vi "MegaAnalysis5.vi"() -> ()   [LabVIEW 2016]
uses:
  <vilib>/Analysis/4window.llb/windowTd.ctl
  <vilib>/Analysis/Matrix/Datatypes/RealMatrix.ctl
  <vilib>/Analysis/baseanly.llb/Mean (DBL).vi
  <vilib>/Analysis/4window.llb/Hanning Window (DBL).vi
  <vilib>/Analysis/2dsp.llb/Real FFT.vi
  <vilib>/Analysis/2dsp.llb/Inverse Real FFT.vi
  <vilib>/Analysis/4window.llb/AllCosWindow (DBL).vi
  subs/status.vi
  <vilib>/Utility/file.llb/Write To Spreadsheet File (I64).vi
  <vilib>/Utility/file.llb/Write To Spreadsheet File (string).vi
  <vilib>/Utility/file.llb/Read From Spreadsheet File (string).vi
  <vilib>/Utility/file.llb/Read From Spreadsheet File (DBL).vi
  <vilib>/Analysis/3filter.llb/Butterworth Filter (DBL).vi
  <vilib>/Analysis/3filter.llb/Chebyshev Filter (DBL).vi
  <vilib>/Analysis/3filter.llb/Inverse Chebyshev Filter (DBL).vi
  <vilib>/Analysis/3filter.llb/Elliptic Filter (DBL).vi
  <vilib>/Analysis/3filter.llb/Bessel Filter (DBL).vi
  <vilib>/measure/mamon.llb/Waveform Peak Detection for 1 Chan.vi
  <vilib>/Analysis/0measdsp.llb/Scaled Time Domain Window (DBL).vi
  <vilib>/Utility/file.llb/Write To Spreadsheet File (DBL).vi
  <vilib>/Analysis/NI_AALBase.lvlib
  <vilib>/measure/NI_MAPro.lvlib
  <vilib>/gmath/NI_Gmath.lvlib
  <vilib>/Analysis/NI_AALPro.lvlib
  <vilib>/Analysis/Matrix/NI_Matrix.lvlib
panel:
  in  "?":bool
  out "activity":string
  in  "?":bool
  in  "transform:":u16(ring)=3 items=["time", "B", "1/B", "data"]
  in  "?":T1(tab)=enum."data select"
  in  "Notes (saved along with settings)":string
  in  "?":bool
  in  "?":bool
  in  "Base path for data storage":path
  in  "?":bool
  in  "?":bool=TRUE
  in  "?":bool=TRUE
  in  "?":bool
  in  "?":bool=TRUE
  in  "?":bool=TRUE
  in  "?":bool
  in  "skip":u16=1
  in  "?":T2(tab)=enum."assign columns"
  in  "files to be imported":path[](array[path])
  in  "?":bool
  out "file contents":string[](array[string])
  in  "?":bool=TRUE
  in  "?":u64=1000
  out "Group name":string="p"
  out "file list":string[][](table)
  out "?":string
  in  "?":bool=TRUE
  in  "column selection options (for each file)":u16(ring) items=["same columns for all files", "different column numbers and scalings"]
  in  "?":T3(tab)=enum."B field"
  in  "clear arrays":bool
  in  "time column rescale":ext[](array[numeric])=[1.0]
  in  "time column selection":u16[](array[numeric])=[0]
  in  "time interval  (for series)":dbl=2e-06 format="%#_6p"
  in  "option":u16(ring) items=["none", "column from file", "create time series"]
  in  "?":bool
  in  "dB/dt column rescale":ext[](array[numeric])=[1.0]
  in  "dB/dt column selection":u16[](array[numeric])=[2]
  in  "option":u16(ring) items=["none", "column from file"]
  in  "clear arrays":bool
  in  "B column selection":u16[](array[numeric])=[0]
  in  "angle theta (cos theta renorm.)":ext[](array[numeric])=[0.0]
  in  "B column rescale":ext[](array[numeric])=[1.0]
  in  "B column offset":ext[](array[numeric])=[0.0]
  in  "clear arrays":bool
  in  "?":dbl
  in  "increment all angles (theta) by:":bool
  in  "read angle from data 2 index:":bool
  in  "?":u32
  in  "?":bool
  in  "?":bool
  in  "?":bool
  in  "?":bool=TRUE
  in  "option":u16(ring)=1 items=["none", "column from file", "1/column from file", "integrate dB/dt"]
  out "time interval":dbl=2e-06 format="%#_6p"
  in  "?":bool=TRUE
  in  "pretrigger time for integration":dbl=0.01 format="%#_6p"
  in  "clear arrays":bool
  in  "divide amplitude rescale amplitude by Sin(2 x angle of B field)":bool
  in  "?":i64=1
  in  "?":bool
  in  "?":bool
  in  "?":bool
  in  "pretrigger time for integration":dbl=0.0001 format="%#_6p"
  in  "data column offset":ext[](array[numeric])=[0.0]
  in  "data column rescale":ext[](array[numeric])=[1.0]
  in  "data column selection":u16[](array[numeric])=[1]
  in  "option":u16(ring)=1 items=["none", "column from file", "1/column from file", "integrate column"]
  out "time interval":dbl=2e-06 format="%#_6p"
  in  "clear arrays":bool
  in  "?":bool
  in  "?":bool
  in  "pretrigger time for integration":dbl=0.0001 format="%#_6p"
  in  "data column offset":ext[](array[numeric])=[0.0]
  in  "data column rescale":ext[](array[numeric])=[1.0]
  in  "data column selection":u16[](array[numeric])=[0]
  in  "option":u16(ring) items=["none", "column from file", "1/column from file", "integrate column"]
  in  "?":bool
  in  "?":i64=100
  out "time interval":dbl=2e-06 format="%#_6p"
  out "# columns":dbl[](array[numeric])
  out "# rows":u64[](array[numeric])
  in  "make all files have same settings as file 0":bool
  in  "upper cutoff":ext
  in  "lower cutoff":ext=32.0
  in  "?":bool
  in  "?":bool=TRUE
  in  "upper cutoff":ext
  in  "lower cutoff":ext
  in  "?":bool
  in  "upper cutoff":u64=1000
  in  "lower cutoff":u64
  in  "?":bool
  in  "mode":bool
  in  "?":T4
  out "file":string="PDOfullsignal4filt"
  in  "file index":u16
  in  "sampling frequency option":u16(ring)=1 items=["determine from time column", "determine from time interval"]
  out "sampling frequency":dbl[](array[numeric])=[1000000.0, 1000000.0]
  in  "left rank":i32=2
  in  "taps":i32=25 min=1
  in  "window":i32(ring)=1 items=["None", "Hanning", "Hamming", "Triangular", "Blackman", "Exact Blackman", "Blackman-Harris", "Kaiser-Bessel", "Flat Top"]
  in  "stopband attenuation (dB)":dbl=60.0 format="%0.2f"
  in  "passband ripple (dB)":dbl=1.0 format="%0.2f"
  in  "attenuation (dB)":dbl=60.0 format="%0.2f"
  in  "ripple(dB)":dbl=0.1 format="%0.2f"
  in  "high cutoff freq: fh":dbl=10000.0 format="%0.2f"
  in  "low cutoff freq: fl":dbl=1000.0 format="%0.4f"
  in  "order":i32=2
  in  "filter type":T5(ring)
  in  "filter selection":u16(ring) items=["none", "Butterworth", "Chebyshev", "Inverse Chebyshev", "Elliptic", "Bessel", "FIR Windowed", "Median"]
  in  "right rank":i32=2
  in  "?":bool
  in  "label":u16(ring) items=["file name", "angle", "temperature"]
  out "?":cluster{"data":ext[], "data":ext[]}[](graph)
  in  "?":bool
  in  "file format":string="%.9f"
  in  "?":bool
  in  "?":u16(ring)=2 items=["extended precision", "double precision", "single precision", "8 bit byte"]
  in  "y axis":u16(ring)=4 items=["Index", "Time", "dB/dt", "B field", "data 1", "data 2"]
  in  "x axis":u16(ring)=3 items=["row", "Time", "dB/dt", "B field", "data 1", "data 2"]
  in  "?":bool
  in  "append name":string=".imp"
  in  "?":bool
  in  "?":T6(tab)=enum."up & down field"
  in  "file name options":u16(ring) items=["keep original file name", "combine first # characters into new name"]
  in  "?":u8=6
  in  "reference option":u16(ring) items=["subtract 1 from 0, 3 from 2, etc. and average dB/dt and B field", "subtract 1 from 0, 3 from 2, etc. and don't average dB/dt and B field", "subtract 0 from 1, 2 from 3, etc. and average dB/dt and B field", "subtract 0 from 1, 2 from 3, etc. and don't average dB/dt and B field"]
  in  "?":bool
  in  "?":u8=6
  in  "?":bool
  in  "append string onto file name":string="ave"
  in  "?":bool
  in  "?":bool
  in  "data options":u16(ring) items=["data 1 only", "data 2 only", "data 1 - data 2", "data 1 + data 2", "magnitude (data 1, 2)"]
  in  "?":dbl
  in  "?":dbl
  in  "?":bool
  in  "?":dbl
  in  "?":bool
  in  "?":dbl
  in  "?":bool
  in  "?":dbl=1.0
  in  "?":bool
  out "file list":string[][](table)
  out "dddd":bool
  in  "field margin for interpolation":dbl=0.2
  in  "field limits:":u16(ring) items=["no field limits", "limit field to within:", "field limits with margins:"]
  in  "minima below :":dbl=100.0
  in  "maxima above:":dbl=5.0
  in  "?":bool=TRUE
  in  "?":cluster{dbl, "and":dbl}[](array[cluster])=[{10.0, "and"=100.0}]
  in  "?":bool=TRUE
  in  "falling sweep start index":dbl[](array[numeric])=[1.0, 2.0, 3.0, 4.0, 5.0, 6.0, 7.0]
  in  "rising sweep start index":dbl[](array[numeric])=[0.0, 1.0, 2.0, 3.0, 4.0, 5.0, 6.0]
  in  "consider variations in B field only above:":dbl=2.0
  out "fields":dbl[][](array[numeric])
  out "row":dbl[][](array[numeric])
  in  "threshold # of points below which field variations are ignored":dbl=100.0
  in  "?":bool
  in  "(slow on large data sets but good for treating small fluctuations in field)":dbl=0.001
  in  "sweeprate-dependent  offset multiplier":dbl
  in  "offset value":dbl
  in  "offset options":u16(ring) items=["none", "constant", "sweeprate sign", "sweeprate dependent"]
  in  "smoothing ratio (must be appreciably larger than 1)":u8=10
  in  "field smoothing":u16(ring) items=["unmodifield", "spline smoothing"]
  in  "label":u16(ring) items=["file name", "angle", "temperature"]
  out "?":cluster{"data":ext[], "data":ext[]}[](graph)
  in  "?":bool
  in  "y axis":u16(ring)=4 items=["Index", "Time", "dB/dt", "B field", "data 1"]
  in  "x axis":u16(ring)=3 items=["row", "Time", "dB/dt", "B field", "data 1"]
  in  "?":bool
  in  "?":bool
  in  "append name":string=".sel"
  in  "saving order":u16(ring) items=["rising first", "falling first"]
  in  "file format":string="%.9f"
  in  "?":u16(ring)=2 items=["extended precision", "double precision", "single precision", "8 bit byte"]
  in  "?":u16(ring)=2 items=["extended precision", "double precision", "single precision", "8 bit byte"]
  in  "?":T7(tab)
  in  "?":bool=TRUE
  in  "rising and falling field options":u16(ring)=5 items=["rising only", "falling only", "sum", "rising - falling", "falling - rising", "greatest # of points"]
  in  "method":i32(ring)=2 items=["nearest", "linear", "spline", "cubic Hermite", "Lagrange"]
  in  "# points":u64=2048
  in  "interpolate in:":u16(ring)=2 items=["time", "B", "1/B", "data"]
  in  "algorithm":T8(ring)=enum."Givens"
  in  "polynomial order":u8=3
  in  "phase":dbl=200.0
  in  "amp":dbl
  in  "F":dbl=200.0
  in  "gamma":dbl=200.0
  in  "special background/filter operations":u16(ring) items=["none", "make oscillations", "subtract oscillations", "oscillation filter", "make time oscillations"]
  in  "post interp amplitude/field modifier":u16(ring) items=["none", "*exp(gamma/B)", "derivative", "2nd derivative", "multiply by Hanning", "background instead of data"]
  in  "background subtraction method":u16(ring)=1 items=["none", "simple subtraction", "divide and subract 1"]
  in  "subtraction type":u16(ring)=1 items=["none", "polynomial fit to data", "polynomial fit to ln(data)", "polynomial fit to 1/data"]
  in  "order":i32=3
  in  "high cutoff":dbl=800.0 format="%0.2f"
  in  "low cutoff":dbl=250.0 format="%0.4f"
  in  "poly sub":dbl=2.0 min=1.0
  out "sampling freq":dbl=226398.48205662225 format="%0.2f"
  in  "filter type":T5(ring)=enum."Bandpass"
  in  "?":bool
  in  "gamma":dbl=200.0
  in  "phase":dbl=200.0
  in  "amp":dbl
  in  "f":dbl=200.0
  in  "gamma":dbl=200.0
  in  "?":bool
  in  "window":T9 items=["Rectangle"=0, "Hanning"=1, "Hamming"=2, "Blackman-Harris"=3, "Exact Blackman"=4, "Blackman"=5, "Flat Top"=6, "4 Term B-Harris "=7, "7 Term B-Harris"=8, "Low Sidelobe"=9, "Blackman Nuttall"=11, "Triangle"=30, "Bartlett-Hanning"=31, "Bohman"=32, "Parzen"=33, "Welch"=34, "Kaiser"=60, "Dolph-Chebyshev"=61, "Gaussian"=62]
  out "?":cluster{"Array 13":ext[], "Array 13":dbl[]}[](graph)
  in  "?":bool
  out "?":cluster{"data":ext[], "Array 13":dbl[]}[](graph)
  out "interpolate in:":u16(ring)=2 items=["time", "B", "1/B", "data"]
  in  "cut off selection":T10(array[cluster])
  in  "?":bool
  in  "?":u8=6
  in  "?":bool
  in  "append string onto file name":string="aveint"
  out "files":string[](array[string])
  in  "label":u16(ring) items=["file name", "angle", "temperature"]
  out "?":cluster{"data":ext[], "data":ext[]}[](graph)
  in  "?":bool
  in  "lower":dbl=60.0
  in  "upper":dbl=20.0
  in  "?":bool
  in  "y axis":u16(ring)=4 items=["time", "dB/dt", "B", "1/B", "data"]
  in  "x axis":u16(ring)=2 items=["time", "dB/dt", "B", "1/B", "data"]
  out "interpolate in:":u16(ring)=2 items=["time", "B", "1/B", "data"]
  in  "?":bool
  in  "?":bool
  in  "append name":string=".int"
  in  "file format":string="%.9f"
  in  "?":bool
  in  "?":T11(tab)
  in  "Increase spectral density":u16(ring)=3 items=["x 1", "x 2", "x 4", "x 8", "x 16", "x 32", "x 64", "x 128", "x 256", "x 512", "x 1024"]
  in  "?":bool
  in  "width":dbl=50.0
  in  "peak finder threshold":dbl=0.05
  in  "truncate spectrum":u16(ring)=4 items=["no", " /2 (nyquist)", "/4", "/8", "/16", "/32", "/64", "/128"]
  in  "padding":u16(ring)=4 items=["x 1", "x 2", "x 4", "x 8", "x 16", "x 32", "x 64", "x 128", "x 256", "x 512", "x 1024"]
  in  "spectrum type":u16(ring) items=["FFT", "maximum entropy"]
  out "interpolate in:":u16(ring)=2 items=["time", "B", "1/B", "data"]
  out "peaks":T12(array[cluster])
  out "files 2":string[](array[string])
  in  "Numeric":dbl
  in  "label":u16(ring) items=["file name", "angle", "temperature"]
  out "?":cluster{"data":ext[], "data":ext[]}[](graph)
  in  "?":u16(ring)=2 items=["extended precision", "double precision", "single precision", "8 bit byte"]
  in  "y axis":u16(ring) items=["amplitude", "power", "phase"]
  in  "?":bool
  in  "?":bool
  in  "file format":string="%.9f"
  in  "append name":string=".fft"
  in  "FT window":T9=1 items=["Rectangle"=0, "Hanning"=1, "Hamming"=2, "Blackman-Harris"=3, "Exact Blackman"=4, "Blackman"=5, "Flat Top"=6, "4 Term B-Harris "=7, "7 Term B-Harris"=8, "Low Sidelobe"=9, "Blackman Nuttall"=11, "Triangle"=30, "Bartlett-Hanning"=31, "Bohman"=32, "Parzen"=33, "Welch"=34, "Kaiser"=60, "Dolph-Chebyshev"=61, "Gaussian"=62]
  in  "Maximum Entropy M":dbl=100.0
  in  "?":enum32{"parameters", "plot"}(tab)=enum."plot"
  out "file list":string[][](table)
  in  "phase":dbl
  in  "amplitude":u16(ring) items=["absolute amplitude", "real component", "imaginary"]
  in  "set B angle as the variable?":bool
  out "mass":dbl[](array[numeric])
  in  "points":u32=100
  in  "interpolation method":i32(ring)=2 items=["nearest", "linear", "spline", "cubic Hermite", "Lagrange"]
  in  "frequencies":dbl[](array[numeric])
  in  "variable (T)":dbl[](array[numeric])
  in  "?":bool
  out "frequencies":cluster{string}[](array[cluster])
  out "?":cluster{dbl[], dbl[]}[](graph)
  in  "?":bool
  in  "?":bool
  in  "file format":string="%.9f"
  in  "append name":string=".amp"
  in  "?":bool=TRUE
  in  "?":u64=1000
  out "file contents":string[](array[string])
  out "saved files":path[](array[path])
  # "\"DO ALL\" list\n(saved with settings)"
  # "rows"
  # "(integration options)"
  # "(integration options)"
  # "OPTIONAL"
  # "dB/dt"
  # "B field"
  # "data 1"
  # "data 2"
  # "row"
  # "time"
  # "OPTIONAL"
  # "all except Median filter"
  # "all except FIR Windowed and Median Filters"
  # "Chebyshev Filter only"
  # "Inverse Chebyshev Filter only"
  # "Elliptic Filter only"
  # "FIR Windowed Filter only"
  # "Median Filter only"
  # "OPTIONAL"
  # "OPTIONAL"
  # "OPTIONAL"
  # "(margins enable interpolation within \nprecise field limits)"
  # "For files in which the field is swept up and down more than once,   rising and falling field sweeps are each numbered 0, 1, 2....... in the order that they occur (i.e. rising field sweeps are each numbered 0, 2, 4....... and falling field sweeps are each numbered 1, 3, 5......  or vice versa)."
  # "detected turning points at which field sweep direction changes"
  # "file & field sweep # associations:"
  # "index"
  # "index"
  # "file #"
  # "file #"
  # "file #"
  # "file #"
  # "OPTIONAL"
  # "(default, unless there are margins in the field limit selection)"
  # "OPTIONAL"
  # "oscillation filter settings (performed w.r.t. interp x)"
  # "make or subtract oscillations settings"
  # "polynomial subtraction settings"
  # "exponential multiplication settings"
  # "make time oscillations settings"
  # "OPTIONAL"
  # "transform"
  # "data"
  # "OPTIONAL"
  # "Maximum Entropy Controls"
  # "FFT controls"
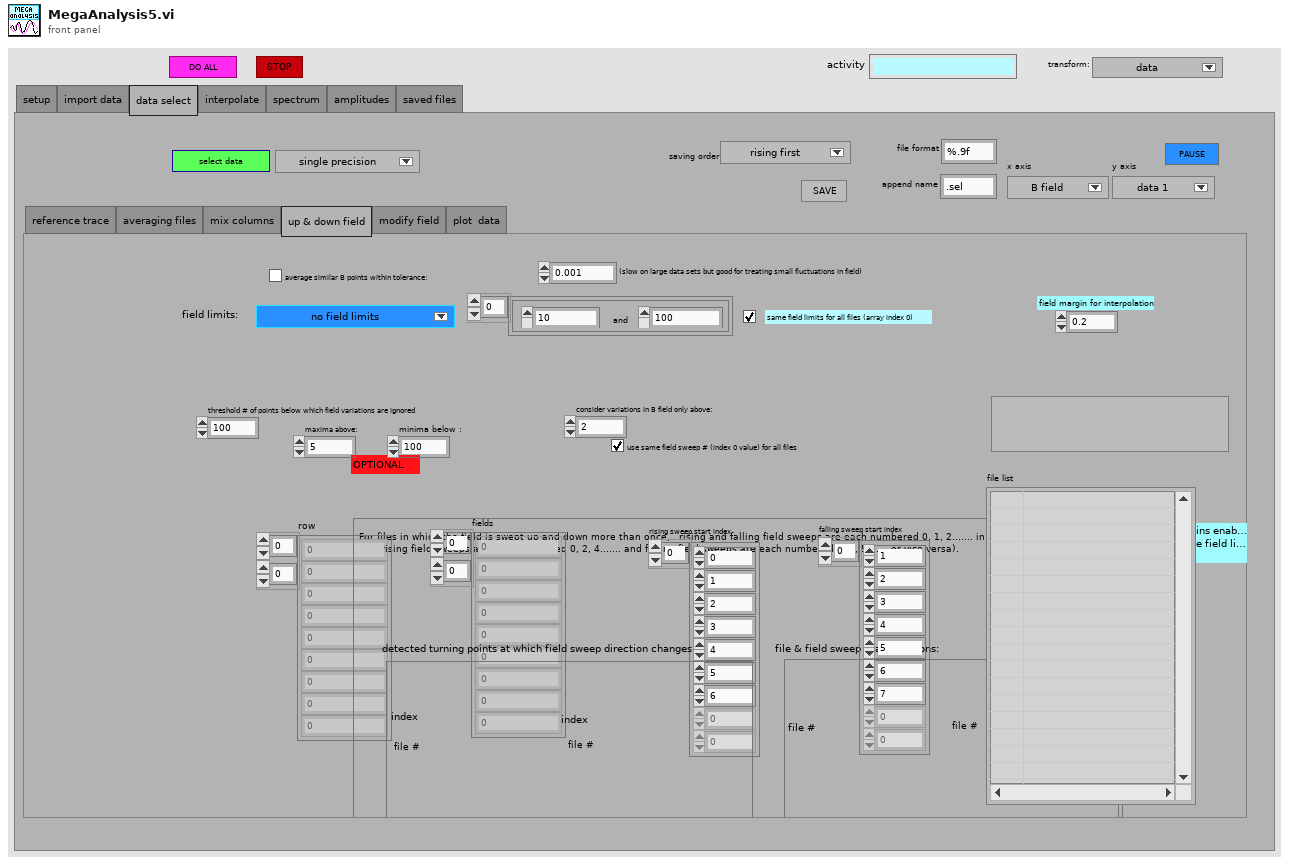
[diagram p1: front panel]
types:
  T1 = enum32{"setup", "import data", "data select", "interpolate", "spectrum", "amplitudes", "saved files"}
  T2 = enum32{"import files", "assign columns", "prescreen data", "edit import", "filter data", "plot import"}
  T3 = enum32{"time", "dB/dt", "B field", "data 1", "data 2"}
  T4 = typedef "NI_Matrix.lvlib/RealMatrix.ctl" = dbl[][]
  T5 = enum32{"Lowpass", "Highpass", "Bandpass", "Bandstop"}
  T6 = enum32{"reference trace", "averaging files", "mix columns", "up & down field", "modify field", "plot  data"}
  T7 = enum32{" options", "background ", "Fourier  filter", "average traces", "plot interpolation"}
  T8 = enum32{"SVD", "Givens", "Givens2", "Householder", "LU Decomposition", "Cholesky"}
  T9 = typedef "NI_AALPro.lvlib/windowTd.ctl" = u32
  T10 = cluster{"lower limit":dbl, "upper limit":dbl, "cuttoff multiplier":dbl}[]
  T11 = enum32{"frequency analysis options", "plot transform"}
  T12 = cluster{"phase":dbl[], "frequency":dbl[], "amplitude":dbl[]}[]
  T13 = cluster{"time column selection ":u16[], "dB/dt column selection":u16[], "B column selection":u16[], "data column selection":u16[], "data column selection":u16[]}
  T14 = cluster{"pretrigger time for integration ":dbl, "pretrigger time for integration ":dbl, "pretrigger time for integration ":dbl}
  T15 = cluster{"time column rescale":ext[], "dB/dt column rescale":ext[], "B column rescale ":ext[], "data column rescale":ext[], "data column rescale":ext[]}
  T16 = cluster{"B column offset":ext[], "data column offset ":ext[], "data column offset":ext[]}
  T17 = typedef "LVCursorListTypeDef.ctl" = cluster{"Name":string, "Color":u32, "Style":u8, "Point Style":u8, "Name Visible":bool, "Allow Drag":bool, "Cursor Mode":u32, "Plot":i32, "Index":i32, "Position":cluster{"X":dbl, "Y":dbl}, "X Scale":u32, "Y Scale":u32, "Watch Plots":i32[], "Watch All Plots":bool, "Plot Area":i32, "Label Offset":cluster{"X":dbl, "Y":dbl}}[]
  T18 = cluster{"Name":string, "Color":u32, "Style":u8, "Point Style":u8, "Name Visible":bool, "Allow Drag":bool, "Cursor Mode":u32, "Plot":i32, "Index":i32, "Position":cluster{"X":dbl, "Y":dbl}, "X Scale":u32, "Y Scale":u32, "Watch Plots":i32[], "Watch All Plots":bool, "Plot Area":i32, "Label Offset":cluster{"X":dbl, "Y":dbl}}
  T19 = cluster{"Value":bool, "Value":bool, "Value":bool, "Value":bool, "Value":bool, "Value":bool}
  T20 = cluster{"Value":u16, "Value":dbl, "Value":u16[], "Value":ext[]}
  T21 = cluster{"Value":u16, "Value":u16[], "Value":ext[], "Value":bool}
  T22 = cluster{"Value":u16, "Value":dbl, "B column selection":u16[], "Value":ext[], "Value":ext[], "Value":ext[], "Value":bool, "Value":bool, "Value":bool, "Value":bool, "Value":u32, "Value":dbl}
  T23 = cluster{"Value":u16, "Value":dbl, "Value":bool, "Value":i64, "Value":u16[], "Value":ext[], "Value":ext[], "Value":bool, "Value":bool}
  T24 = cluster{"Value":u16, "Value":bool, cluster{"Value":u16, "Value":dbl, "Value":u16[], "Value":ext[]}, cluster{"Value":u16, "Value":u16[], "Value":ext[], "Value":bool}, cluster{"Value":u16, "Value":dbl, "B column selection":u16[], "Value":ext[], "Value":ext[], "Value":ext[], "Value":bool, "Value":bool, "Value":bool, "Value":bool, "Value":u32, "Value":dbl}, cluster{"Value":u16, "Value":dbl, "Value":bool, "Value":i64, "Value":u16[], "Value":ext[], "Value":ext[], "Value":bool, "Value":bool}, cluster{"Value":u16, "Value":dbl, "Value":bool, "Value":i64, "Value":u16[], "Value":ext[], "Value":ext[], "Value":bool, "Value":bool}}
  T25 = cluster{"Value":bool, "Value":bool, "Value":bool, "Value":u64, "Value":ext, "Value":ext, "Value":u64, "Value":ext, "Value":ext, "Value":bool}
  T26 = cluster{"Value":u16, "Value":u16, "Value":dbl[], "Value":enum32{"Lowpass", "Highpass", "Bandpass", "Bandstop"}, "Value":dbl, "Value":dbl, "Value":i32, "Value":dbl, "Value":dbl, "Value":dbl, "Value":i32, "Value":i32, "Value":i32, "Value":i32, "Value":dbl}
  T27 = cluster{"Value":path[], cluster{"Value":u16, "Value":bool, cluster{"Value":u16, "Value":dbl, "Value":u16[], "Value":ext[]}, cluster{"Value":u16, "Value":u16[], "Value":ext[], "Value":bool}, cluster{"Value":u16, "Value":dbl, "B column selection":u16[], "Value":ext[], "Value":ext[], "Value":ext[], "Value":bool, "Value":bool, "Value":bool, "Value":bool, "Value":u32, "Value":dbl}, cluster{"Value":u16, "Value":dbl, "Value":bool, "Value":i64, "Value":u16[], "Value":ext[], "Value":ext[], "Value":bool, "Value":bool}, cluster{"Value":u16, "Value":dbl, "Value":bool, "Value":i64, "Value":u16[], "Value":ext[], "Value":ext[], "Value":bool, "Value":bool}}, cluster{"Value":bool, "Value":bool, "Value":bool, "Value":u64, "Value":ext, "Value":ext, "Value":u64, "Value":ext, "Value":ext, "Value":bool}, cluster{"Value":u16, "Value":u16, "Value":dbl[], "Value":enum32{"Lowpass", "Highpass", "Bandpass", "Bandstop"}, "Value":dbl, "Value":dbl, "Value":i32, "Value":dbl, "Value":dbl, "Value":dbl, "Value":i32, "Value":i32, "Value":i32, "Value":i32, "Value":dbl}, cluster{"Value":string, "Value":bool}}
  T28 = cluster{"Value":u16, "Value":u16, "Value":string, cluster{"Value":path[], cluster{"Value":u16, "Value":bool, cluster{"Value":u16, "Value":dbl, "Value":u16[], "Value":ext[]}, cluster{"Value":u16, "Value":u16[], "Value":ext[], "Value":bool}, cluster{"Value":u16, "Value":dbl, "B column selection":u16[], "Value":ext[], "Value":ext[], "Value":ext[], "Value":bool, "Value":bool, "Value":bool, "Value":bool, "Value":u32, "Value":dbl}, cluster{"Value":u16, "Value":dbl, "Value":bool, "Value":i64, "Value":u16[], "Value":ext[], "Value":ext[], "Value":bool, "Value":bool}, cluster{"Value":u16, "Value":dbl, "Value":bool, "Value":i64, "Value":u16[], "Value":ext[], "Value":ext[], "Value":bool, "Value":bool}}, cluster{"Value":bool, "Value":bool, "Value":bool, "Value":u64, "Value":ext, "Value":ext, "Value":u64, "Value":ext, "Value":ext, "Value":bool}, cluster{"Value":u16, "Value":u16, "Value":dbl[], "Value":enum32{"Lowpass", "Highpass", "Bandpass", "Bandstop"}, "Value":dbl, "Value":dbl, "Value":i32, "Value":dbl, "Value":dbl, "Value":dbl, "Value":i32, "Value":i32, "Value":i32, "Value":i32, "Value":dbl}, cluster{"Value":string, "Value":bool}}}
  T29 = cluster{"Value":bool, "Value":u16, "Value":u16, "Value":u8}
  T30 = cluster{"Value":bool, "Value":string, "Value":bool, "Value":u8}
  T31 = cluster{"Value":u16, "Value":bool, "Value":dbl, "Value":bool, "Value":dbl, "Value":bool, "Value":dbl, "Value":bool, "Value":dbl, "Value":bool, "Value":dbl}
  T32 = cluster{"Value":bool, "Value":dbl, "Value":u16, "Value":cluster{dbl, "and":dbl}[], "Value":bool, "Value":dbl, "Value":dbl, "Value":bool, "Value":dbl[][], "Value":dbl[][], "Value":dbl[], "Value":dbl[], "Value":dbl, "Value":dbl}
  T33 = cluster{"Value":u16, "Value":u8, "Value":u16, "Value":dbl, "Value":dbl}
  T34 = cluster{cluster{"Value":bool, "Value":u16, "Value":u16, "Value":u8}, cluster{"Value":bool, "Value":string, "Value":bool, "Value":u8}, cluster{"Value":u16, "Value":bool, "Value":dbl, "Value":bool, "Value":dbl, "Value":bool, "Value":dbl, "Value":bool, "Value":dbl, "Value":bool, "Value":dbl}, cluster{"Value":bool, "Value":dbl, "Value":u16, "Value":cluster{dbl, "and":dbl}[], "Value":bool, "Value":dbl, "Value":dbl, "Value":bool, "Value":dbl[][], "Value":dbl[][], "Value":dbl[], "Value":dbl[], "Value":dbl, "Value":dbl}, "Value":string, cluster{"Value":u16, "Value":u8, "Value":u16, "Value":dbl, "Value":dbl}}
  T35 = cluster{"Value":u16, cluster{cluster{"Value":bool, "Value":u16, "Value":u16, "Value":u8}, cluster{"Value":bool, "Value":string, "Value":bool, "Value":u8}, cluster{"Value":u16, "Value":bool, "Value":dbl, "Value":bool, "Value":dbl, "Value":bool, "Value":dbl, "Value":bool, "Value":dbl, "Value":bool, "Value":dbl}, cluster{"Value":bool, "Value":dbl, "Value":u16, "Value":cluster{dbl, "and":dbl}[], "Value":bool, "Value":dbl, "Value":dbl, "Value":bool, "Value":dbl[][], "Value":dbl[][], "Value":dbl[], "Value":dbl[], "Value":dbl, "Value":dbl}, "Value":string, cluster{"Value":u16, "Value":u8, "Value":u16, "Value":dbl, "Value":dbl}}}
  T36 = cluster{"Value":u16, "Value":u64, "Value":i32, "Value":u16, "Value":bool}
  T37 = cluster{"Value":u16, "Value":u16, "Value":u16, "Value":u16, "Value":bool, "Value":enum32{"Lowpass", "Highpass", "Bandpass", "Bandstop"}, "Value":dbl, "Value":dbl, "Value":dbl, "Value":dbl, "Value":i32, "Value":dbl, "Value":dbl, "Value":dbl, "Value":dbl, "Value":enum32{"SVD", "Givens", "Givens2", "Householder", "LU Decomposition", "Cholesky"}, "Value":u8, "Value":dbl, "Value":dbl, "Value":dbl, "Value":dbl, "Value":dbl}
  T38 = cluster{"Value":bool, "Value":cluster{"lower limit":dbl, "upper limit":dbl, "cuttoff multiplier":dbl}[], "Value":T9}
  T39 = cluster{"Value":bool, "Value":dbl, "Value":dbl, "Value":string}
  T40 = cluster{cluster{"Value":u16, "Value":u64, "Value":i32, "Value":u16, "Value":bool}, cluster{"Value":u16, "Value":u16, "Value":u16, "Value":u16, "Value":bool, "Value":enum32{"Lowpass", "Highpass", "Bandpass", "Bandstop"}, "Value":dbl, "Value":dbl, "Value":dbl, "Value":dbl, "Value":i32, "Value":dbl, "Value":dbl, "Value":dbl, "Value":dbl, "Value":enum32{"SVD", "Givens", "Givens2", "Householder", "LU Decomposition", "Cholesky"}, "Value":u8, "Value":dbl, "Value":dbl, "Value":dbl, "Value":dbl, "Value":dbl}, cluster{"Value":bool, "Value":cluster{"lower limit":dbl, "upper limit":dbl, "cuttoff multiplier":dbl}[], "Value":T9}, cluster{"Value":bool, "Value":string, "Value":bool, "Value":u8}, cluster{"Value":bool, "Value":dbl, "Value":dbl, "Value":string}}
  T41 = cluster{"Value":u16, cluster{cluster{"Value":u16, "Value":u64, "Value":i32, "Value":u16, "Value":bool}, cluster{"Value":u16, "Value":u16, "Value":u16, "Value":u16, "Value":bool, "Value":enum32{"Lowpass", "Highpass", "Bandpass", "Bandstop"}, "Value":dbl, "Value":dbl, "Value":dbl, "Value":dbl, "Value":i32, "Value":dbl, "Value":dbl, "Value":dbl, "Value":dbl, "Value":enum32{"SVD", "Givens", "Givens2", "Householder", "LU Decomposition", "Cholesky"}, "Value":u8, "Value":dbl, "Value":dbl, "Value":dbl, "Value":dbl, "Value":dbl}, cluster{"Value":bool, "Value":cluster{"lower limit":dbl, "upper limit":dbl, "cuttoff multiplier":dbl}[], "Value":T9}, cluster{"Value":bool, "Value":string, "Value":bool, "Value":u8}, cluster{"Value":bool, "Value":dbl, "Value":dbl, "Value":string}}}
  T42 = cluster{"Value":u16, "Value":u16, "Value":bool, "Value":dbl, "Value":u16, "Value":u16, "Value":u16, "Value":dbl}
  T43 = cluster{cluster{"Value":u16, "Value":u16, "Value":bool, "Value":dbl, "Value":u16, "Value":u16, "Value":u16, "Value":dbl}, cluster{"Value":T9, "Value":dbl, "Value":string}}
  T44 = cluster{"Value":u16, cluster{cluster{"Value":u16, "Value":u16, "Value":bool, "Value":dbl, "Value":u16, "Value":u16, "Value":u16, "Value":dbl}, cluster{"Value":T9, "Value":dbl, "Value":string}}}
  T45 = cluster{"Value":dbl[], "Value":bool, "Value":u32, "Value":dbl[], "Value":i32, "Value":u16, "Value":dbl}
  T46 = cluster{cluster{"Value":dbl[], "Value":bool, "Value":u32, "Value":dbl[], "Value":i32, "Value":u16, "Value":dbl}, "Value":string}
  T47 = cluster{cluster{"Value":bool, "Value":bool, "Value":bool, "Value":bool, "Value":bool, "Value":bool}, cluster{"Value":u16, "Value":u16, "Value":string, cluster{"Value":path[], cluster{"Value":u16, "Value":bool, cluster{"Value":u16, "Value":dbl, "Value":u16[], "Value":ext[]}, cluster{"Value":u16, "Value":u16[], "Value":ext[], "Value":bool}, cluster{"Value":u16, "Value":dbl, "B column selection":u16[], "Value":ext[], "Value":ext[], "Value":ext[], "Value":bool, "Value":bool, "Value":bool, "Value":bool, "Value":u32, "Value":dbl}, cluster{"Value":u16, "Value":dbl, "Value":bool, "Value":i64, "Value":u16[], "Value":ext[], "Value":ext[], "Value":bool, "Value":bool}, cluster{"Value":u16, "Value":dbl, "Value":bool, "Value":i64, "Value":u16[], "Value":ext[], "Value":ext[], "Value":bool, "Value":bool}}, cluster{"Value":bool, "Value":bool, "Value":bool, "Value":u64, "Value":ext, "Value":ext, "Value":u64, "Value":ext, "Value":ext, "Value":bool}, cluster{"Value":u16, "Value":u16, "Value":dbl[], "Value":enum32{"Lowpass", "Highpass", "Bandpass", "Bandstop"}, "Value":dbl, "Value":dbl, "Value":i32, "Value":dbl, "Value":dbl, "Value":dbl, "Value":i32, "Value":i32, "Value":i32, "Value":i32, "Value":dbl}, cluster{"Value":string, "Value":bool}}}, cluster{"Value":u16, cluster{cluster{"Value":bool, "Value":u16, "Value":u16, "Value":u8}, cluster{"Value":bool, "Value":string, "Value":bool, "Value":u8}, cluster{"Value":u16, "Value":bool, "Value":dbl, "Value":bool, "Value":dbl, "Value":bool, "Value":dbl, "Value":bool, "Value":dbl, "Value":bool, "Value":dbl}, cluster{"Value":bool, "Value":dbl, "Value":u16, "Value":cluster{dbl, "and":dbl}[], "Value":bool, "Value":dbl, "Value":dbl, "Value":bool, "Value":dbl[][], "Value":dbl[][], "Value":dbl[], "Value":dbl[], "Value":dbl, "Value":dbl}, "Value":string, cluster{"Value":u16, "Value":u8, "Value":u16, "Value":dbl, "Value":dbl}}}, cluster{"Value":u16, cluster{cluster{"Value":u16, "Value":u64, "Value":i32, "Value":u16, "Value":bool}, cluster{"Value":u16, "Value":u16, "Value":u16, "Value":u16, "Value":bool, "Value":enum32{"Lowpass", "Highpass", "Bandpass", "Bandstop"}, "Value":dbl, "Value":dbl, "Value":dbl, "Value":dbl, "Value":i32, "Value":dbl, "Value":dbl, "Value":dbl, "Value":dbl, "Value":enum32{"SVD", "Givens", "Givens2", "Householder", "LU Decomposition", "Cholesky"}, "Value":u8, "Value":dbl, "Value":dbl, "Value":dbl, "Value":dbl, "Value":dbl}, cluster{"Value":bool, "Value":cluster{"lower limit":dbl, "upper limit":dbl, "cuttoff multiplier":dbl}[], "Value":T9}, cluster{"Value":bool, "Value":string, "Value":bool, "Value":u8}, cluster{"Value":bool, "Value":dbl, "Value":dbl, "Value":string}}}, cluster{"Value":u16, cluster{cluster{"Value":u16, "Value":u16, "Value":bool, "Value":dbl, "Value":u16, "Value":u16, "Value":u16, "Value":dbl}, cluster{"Value":T9, "Value":dbl, "Value":string}}}, cluster{cluster{"Value":dbl[], "Value":bool, "Value":u32, "Value":dbl[], "Value":i32, "Value":u16, "Value":dbl}, "Value":string}, "Notes (saved along with settings)":string}
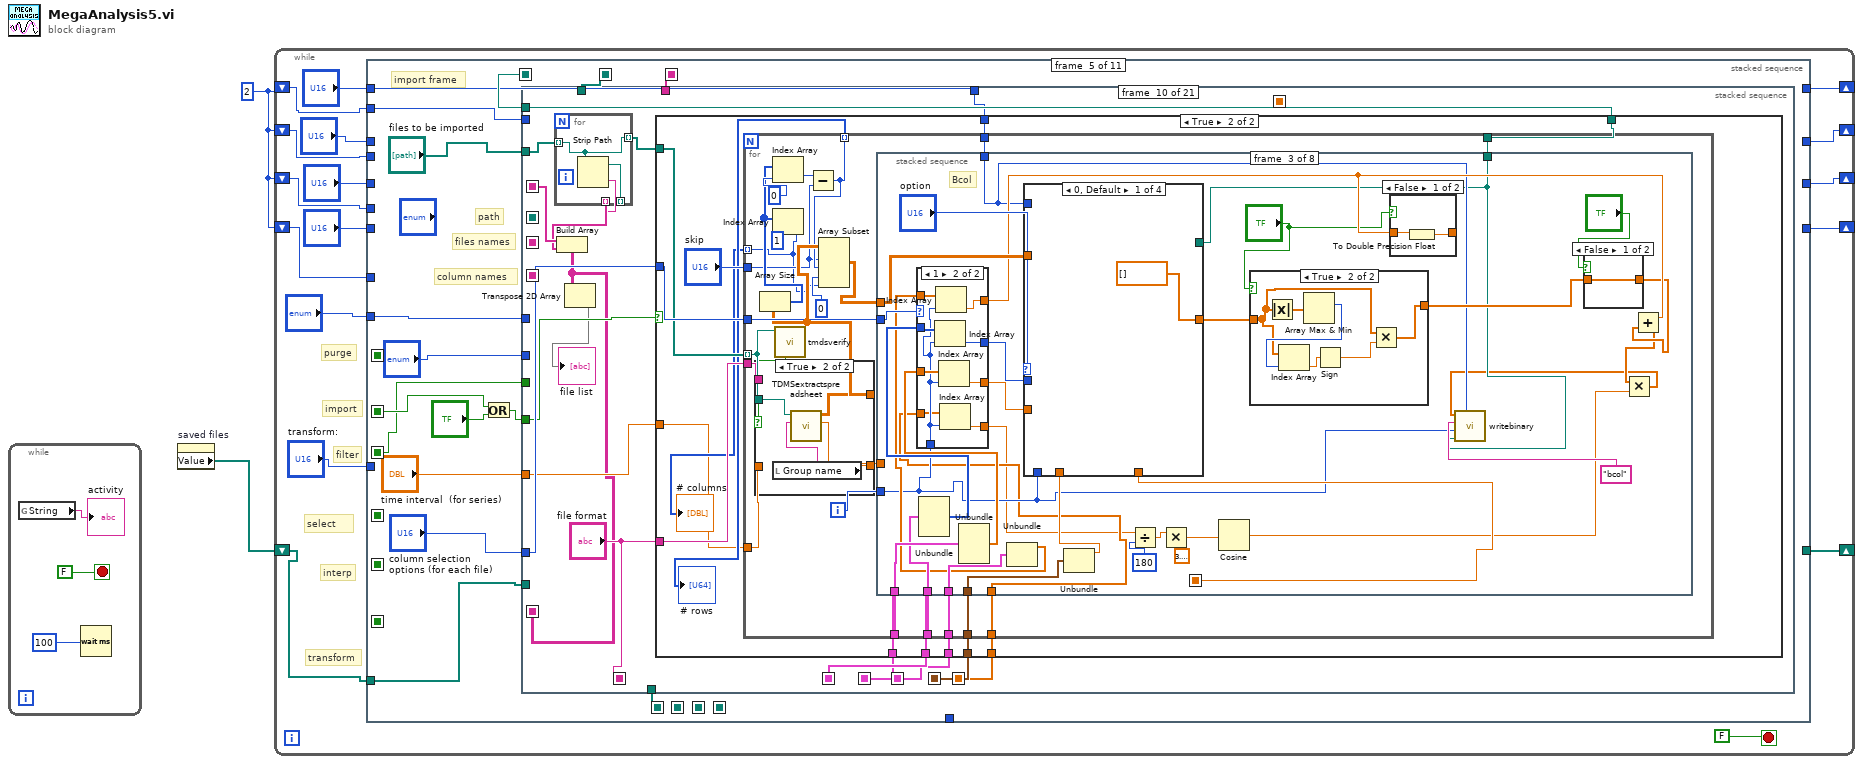
[diagram p0: block diagram]
diagram:
  w2 = 2
  n1 = while {
    stop <- FALSE stop-if-true
    n2 = global read "status.vi" "String"() -> (→"activity":string)
    n3 = Wait (ms)(milliseconds to wait=100) -> ()  [unwired: 1 out]
  }
  n4 = property on="saved files" class="Arr (strict)"() -> ("Value"=w1:path[])  [unwired: 2 in, 2 out]
  n5 = while {
    shift-right: [w16] -> _
    shift-left: w2 -> [w12]
    shift-right: [w15] -> _
    shift-left: w2 -> [w11]
    shift-right: [w14] -> _
    shift-left: w2 -> [w10]
    shift-right: [w13] -> _
    shift-left: w2 -> [w9]
    shift-right: [w6] -> _
    shift-left: w1 -> [w7]
    stop <- FALSE stop-if-true
    # "transform"
    # "interp"
    # "select"
    # "filter"
    # "import"
    # "purge"
    n6 = stacked-sequence {
      seq-local: [w23 _ _ _ _ _ _ _ _ _ _] -> [_ _ w101 w126 w157 w1417 w3251 w4640 w5014 _ _]
      seq-local: [_ _ _ _ w156 _ _ _ _ _ _] -> [_ _ _ _ _ _ _ _ _ _ _]
      seq-local: [_ _ _ _ w155 _ _ _ _ _ _] -> [_ _ _ _ _ _ _ _ _ _ _]
      seq-local: [_ w63 _ _ _ _ _ _ _ _ _] -> [_ _ _ w124 _ _ _ _ _ _ _]
      seq-local: [_ w62 _ _ _ _ _ _ _ _ _] -> [_ _ _ _ w149 _ _ _ _ _ _]
      seq-local: [_ w61 _ _ _ _ _ _ _ _ _] -> [_ _ _ _ w148 _ _ _ _ _ _]
      seq-local: [_ w60 _ _ _ _ _ _ _ _ _] -> [_ _ _ _ _ w1403 _ _ _ _ _]
      seq-local: [_ w59 _ _ _ _ _ _ _ _ _] -> [_ _ _ _ _ _ w3240 _ _ _ _]
      seq-local: [_ w58 _ _ _ _ _ _ _ _ _] -> [_ _ _ _ _ _ _ w4630 _ _ _]
      seq-local: [_ _ _ _ w146 _ _ _ _ _ _] -> [_ _ _ _ _ w1402 _ _ _ _ _]
      seq-local: [_ _ _ _ _ w1401 _ _ _ _ _] -> [_ _ _ _ _ _ w3239 _ _ _ _]
      seq-local: [_ _ _ _ _ _ w3238 _ _ _ _] -> [_ _ _ _ _ _ _ w4629 _ _ _]
      seq-local: [_ _ _ _ _ _ _ w4628 _ _ _] -> [_ _ _ _ _ _ _ _ w5022 _ _]
      tunnel: "?" -> [_ w56 _ _ w160 w1416 w3249 w4635 w5030 _ _]
      tunnel: "transform:" -> [_ _ _ _ _ _ w3246 w4639 _ _ _]
      tunnel: "?" -> [_ w73 _ _ w154 w1408 _ _ _ _ _]
      tunnel: "?" -> [_ w72 _ _ _ w1407 w3244 _ _ _ _]
      tunnel: "?" -> [_ w71 _ _ _ _ w3245 w4634 w5023 _ _]
      tunnel: "?" -> [_ w70 _ _ _ _ _ w4633 w5036 _ _]
      tunnel: [_ w73 _ _ _ _ _ _ _ _ _] -> w16
      tunnel: [_ w72 _ _ _ _ _ _ _ _ _] -> w15
      tunnel: [_ w71 _ _ _ _ _ _ _ _ _] -> w14
      tunnel: [_ w70 _ _ _ _ _ _ _ _ _] -> w13
      tunnel: w12 -> [_ _ _ _ w153 _ _ _ _ _ _]
      tunnel: w11 -> [_ _ _ _ _ w1406 _ _ _ _ _]
      tunnel: w10 -> [_ _ _ _ _ _ w3243 _ _ _ _]
      tunnel: w9 -> [_ _ _ _ _ _ _ w4632 _ _ _]
      tunnel: w7 -> [_ w55 _ _ w147 _ _ _ _ _ _]
      tunnel: [_ _ _ _ _ _ _ _ w5021 _ _] -> w6
      tunnel: [_ _ _ _ _ _ _ _ _ _ w5779] -> _
      frame #0 {
        n7 = stacked-sequence {
          tunnel: [w35] -> w24
          frame #0 {
            n8 = Empty String/Path?(string/path="Base path for data storage") -> (empty?=w30:bool)
            n9 = Current VI's Path() -> (path=w34:path)
            n10 = Not(x=w30) -> (.not. x?=w29:bool)
            n11 = call <vilib>:"Check if File or Folder Exists.vi"("path"="Base path for data storage") -> ("file or folder exists?"=w32:bool)  [unwired: 1 in, 9 out]
            n12 = Strip Path(path=w34) -> (stripped path=w33:path)  [unwired: 1 out]
            n13 = And(x=w32, y=w29) -> (x .and. y?=w31:bool)
            n14 = case shown="False" w31 {
              tunnel: [w37 w48] -> w35
              tunnel: "Base path for data storage" -> [_ w49]
              tunnel: w33 -> [w36 _]
              frame False {
                n15 = disable-structure shown="Enabled" {
                  disable-tunnel: [w41 w44] -> w39
                  disable-tunnel: [w40 w45] -> w38
                  frame Disabled {
                    n16 = Create Folder(prompt (Create Folder)="Create folder for temporary data storage") -> (created path=w40:path, cancelled=w41:bool)  [unwired: 2 in, 1 out]
                  }
                  frame Enabled {
                    n17 = call "File Dialog"("prompt"="Select or create folder for temporary data storage") -> ("selected path"=w45:path, "cancelled"=w44:bool)  [unwired: 11 in, 2 out]
                  }
                }
                n18 = case shown="True" w39 {
                  tunnel: w38 -> [w46 _]
                  tunnel: [w46 w47] -> w37
                  tunnel: w36 -> [_ w47]
                  frame False {
                  }
                  frame True {
                  }
                }
              }
              frame True {
                n19 = Strip Path(path=w49) -> (stripped path=w48:path)  [unwired: 1 out]
              }
            }
          }
        }
        n20 = Build Path(base path=w24, name or relative path="data") -> (appended path=w23:path)
        n21 = call <vilib>:"Check if File or Folder Exists.vi"("path"=w23) -> ("file or folder exists?"=w26:bool, "dup path"=w25:path)  [unwired: 1 in, 8 out]
        n22 = local write "Base path for data storage"(w23) -> ()
        n23 = case shown="True" w26 {
          tunnel: w25 -> [w50 _]
          frame False {
            n24 = Create Folder(path (use dialog)=w50) -> ()  [unwired: 1 in, 4 out]
          }
          frame True {
          }
        }
      }
      frame #1 {
        # "setup frame"
        n25 = And(x="?", y="?") -> (x .and. y?=w59:bool)
        n26 = And(x="?", y="?") -> (x .and. y?=w60:bool)
        n27 = And(x="?", y="?") -> (x .and. y?=w58:bool)
        n28 = And(x="?", y="?") -> (x .and. y?=w61:bool)
        n29 = And(x="?", y="?") -> (x .and. y?=w62:bool)
        n30 = And(x="?", y="?") -> (x .and. y?=w63:bool)
        n31 = Equal?(x=w56, y=6) -> (x = y?=w54:bool)
        n32 = global write "status.vi" "String"("front panel") -> ()
        n33 = for {
          tunnel: w54 -> [w76]
          tunnel: [w75] -> w53 mode=indexing
          tunnel: w55 -> [w74] mode=indexing
          n34 = stacked-sequence {
            tunnel: w76 -> [w79]
            tunnel: w74 -> [w80]
            tunnel: [w81] -> w75
            frame #0 {
              n35 = Empty String/Path?(string/path=w80) -> (empty?=w82:bool)
              n36 = case shown="True" w79 {
                tunnel: ["" w88] -> w81
                tunnel: w82 -> [_ w87]
                tunnel: w80 -> [_ w86]
                tunnel: "?" -> [_ w85]
                tunnel: "?" -> [_ w84]
                frame False {
                }
                frame True {
                  n37 = case shown="False" w87 {
                    tunnel: [w92 ""] -> w88
                    tunnel: w86 -> [w91 _]
                    tunnel: w85 -> [w90 _]
                    tunnel: w84 -> [w89 _]
                    frame False {
                      n38 = case shown="True" w90 {
                        tunnel: [w94 w95] -> w92
                        tunnel: w91 -> [w93 w99]
                        tunnel: w89 -> [_ w98]
                        frame False {
                          n39 = Read from Text File(file (use dialog)=w93) -> (text=w94:string)  [unwired: 2 in, 4 out]
                        }
                        frame True {
                          n40 = Read from Text File(file (use dialog)=w99) -> (text=w96:string)  [unwired: 2 in, 4 out]
                          n41 = String Subset(string=w96, offset (0)=0, length (rest)=w98) -> (substring=w95:string)
                        }
                      }
                    }
                    frame True {
                    }
                  }
                }
              }
            }
          }
        }
        "file contents" <- w53
        "saved files" <- w55
      }
      frame #2 {
        # "setup frame 2"
        n42 = Build Array("files", "files2", "files3", "files4", "paths", "paths2", "paths3", "paths4") -> (w109:string[])
        n43 = for {
          tunnel: w109 -> [w120] mode=indexing
          tunnel: w101 -> [w117]
          n44 = Build Path(base path=w117, name or relative path=w120) -> (appended path=w118:path)
          n45 = call <vilib>:"Check if File or Folder Exists.vi"("path"=w118) -> ("file or folder exists?"=w119:bool)  [unwired: 1 in, 9 out]
          n46 = case shown="False" w119 {
            tunnel: w118 -> [w122 _]
            frame False {
              n47 = call-poly <vilib>:"Write To Spreadsheet File.vi"("1D data"=string[] [] ("Array 17"), "file path (dialog if empty)"=w122) -> ()  [unwired: 4 in, 3 out]
            }
            frame True {
            }
          }
        }
        n48 = Build Path(base path=w101, name or relative path="filecount") -> (appended path=w103:path)
        n49 = call <vilib>:"Check if File or Folder Exists.vi"("path"=w103) -> ("file or folder exists?"=w102:bool)  [unwired: 1 in, 9 out]
        n50 = case shown="False" w102 {
          tunnel: w103 -> [w116 _]
          frame False {
            n51 = Build Array(0) -> (w114:i32[])
            n52 = call-poly <vilib>:"Write To Spreadsheet File.vi"("1D data"=w114, "file path (dialog if empty)"=w116) -> ()  [unwired: 4 in, 3 out]
          }
          frame True {
          }
        }
      }
      frame #3 {
        # "purge frame"
        n53 = Or(x=w124, y="?") -> (x .or. y?=w123:bool)
        n54 = case shown="True" w123 {
          tunnel: w126 -> [_ w131]
          frame False {
          }
          frame True {
            n55 = Build Array("files", "files2", "files3", "files4", "paths", "paths2", "paths3", "paths4", "table", "tfits", "afits") -> (w136:string[])
            n56 = for {
              tunnel: w136 -> [w143] mode=indexing
              tunnel: w131 -> [w144]
              n57 = Build Path(base path=w144, name or relative path=w143) -> (appended path=w142:path)
              n58 = call-poly <vilib>:"Write To Spreadsheet File.vi"("1D data"=string[] [] ("Array 4"), "file path (dialog if empty)"=w142) -> ()  [unwired: 4 in, 3 out]
            }
            n59 = global write "status.vi" "String"("purging") -> ()
          }
        }
      }
      frame #4 {
        # "import frame"
        # "path"
        # "column names"
        # "files names"
        n60 = Or(x=w149, y="?") -> (x .or. y?=w151:bool)
        n61 = stacked-sequence {
          seq-local: [_ _ w244 _ _ _ _ _ _ _ _ _ _ _ _ _ _ _ _ _ _] -> [_ _ _ _ _ _ _ _ _ w376 _ _ _ _ _ _ _ _ _ _ _]
          seq-local: [_ _ w243 _ _ _ _ _ _ _ _ _ _ _ _ _ _ _ _ _ _] -> [_ _ _ _ _ _ _ _ w343 w375 _ _ _ _ _ _ _ _ _ _ _]
          seq-local: [_ _ w239 _ _ _ _ _ _ _ _ _ _ _ _ _ _ _ _ _ _] -> [_ _ _ _ _ _ _ _ _ w372 _ _ _ _ _ _ _ _ _ _ _]
          seq-local: [_ _ w235 _ _ _ _ _ _ _ _ _ _ _ _ _ _ _ _ _ _] -> [_ _ _ _ _ _ _ _ _ w371 _ _ _ _ _ _ _ _ _ _ _]
          seq-local: [_ _ _ _ _ w282 _ _ _ _ _ _ _ _ _ _ _ _ _ _ _] -> [_ _ _ _ _ _ w293 _ _ _ w844 _ w940 w965 w989 w1033 w1100 w1152 w1201 _ w1389]
          seq-local: [_ _ _ _ w272 _ _ _ _ _ _ _ _ _ _ _ _ _ _ _ _] -> [_ _ _ _ _ _ w291 _ _ _ _ _ _ w964 w988 w1032 w1102 w1162 w1200 _ _]
          seq-local: [_ _ _ _ _ w280 _ _ _ _ _ _ _ _ _ _ _ _ _ _ _] -> [_ _ _ _ _ _ _ _ _ _ _ _ _ _ _ _ _ _ w1202 _ w1390]
          seq-local: [_ _ _ _ _ _ _ _ _ "file format" _ _ _ _ _ _ _ _ _ _ _] -> [_ _ _ _ _ _ _ _ _ _ _ _ _ _ _ _ _ _ w1203 _ _]
          seq-local: [_ _ _ _ _ _ _ _ _ _ _ _ w938 _ _ _ _ _ _ _ _] -> [_ _ _ _ _ _ _ _ _ _ _ _ _ _ _ _ _ _ _ w1258 _]
          seq-local: [_ _ w225 _ _ _ _ _ _ _ _ _ _ _ _ _ _ _ _ _ _] -> [_ _ _ _ _ _ _ _ w341 w366 _ _ _ _ _ _ _ _ _ _ _]
          seq-local: [w162 _ _ _ _ _ _ _ _ _ _ _ _ _ _ _ _ _ _ _ _] -> [_ _ _ _ _ _ _ _ _ w365 _ _ _ _ _ _ _ _ _ _ _]
          seq-local: [_ _ _ _ _ _ _ _ _ w362 _ _ _ _ _ _ _ _ _ _ _] -> [_ _ _ _ _ _ _ _ _ _ _ _ _ _ _ _ _ _ _ _ _]
          tunnel: w160 -> [_ w176 _ _ _ _ _ _ _ _ _ _ _ _ _ _ w1099 w1160 _ _ _]
          tunnel: "?" -> [_ w175 _ _ _ _ _ _ _ _ _ _ _ _ _ _ w1103 w1164 _ _ _]
          tunnel: "files to be imported" -> [w165 w174 _ w258 _ _ _ _ _ w374 _ w857 _ _ _ _ _ _ _ _ _]
          tunnel: "column selection options (for each file)" -> [w168 _ _ _ _ _ _ _ _ w378 _ _ _ _ _ _ _ _ _ _ _]
          tunnel: w157 -> [_ _ _ w256 _ w279 w292 _ _ w377 w842 _ w939 w963 w990 w1034 w1101 w1161 w1204 w1263 w1391]
          tunnel: [_ _ _ _ _ _ _ _ _ _ _ _ _ _ _ _ _ _ w1202 _ _] -> w156
          tunnel: [_ _ _ _ _ _ _ _ _ _ _ _ _ _ _ _ _ _ w1200 _ _] -> w155
          tunnel: w151 -> [w161 _ _ w257 _ _ _ _ _ w369 _ _ _ w960 w986 w1031 _ _ _ _ w1392]
          tunnel: w154 -> [_ _ _ _ _ _ w288 _ _ w368 w843 _ w937 w959 w984 w1028 w1096 w1157 w1199 w1257 _]
          tunnel: w153 -> [_ _ _ _ _ _ w287 _ _ _ _ _ _ _ _ _ _ _ _ _ _]
          tunnel: "time interval  (for series)" -> [w166 _ _ _ _ _ _ _ _ w367 _ _ w935 _ _ _ _ _ _ _ _]
          tunnel: w148 -> [_ _ _ _ _ _ _ _ _ _ _ _ _ _ _ _ _ _ _ w1254 _]
          tunnel: w147 -> [_ _ _ _ _ _ _ _ _ _ _ _ _ _ _ _ _ _ w1198 _ _]
          tunnel: [_ _ _ _ _ _ _ _ _ _ _ _ _ _ _ _ _ _ w1197 _ _] -> w146
          frame #0 {
            n62 = for {
              tunnel: w165 -> [_] mode=indexing
              tunnel: [w170] -> w164 mode=indexing
              i -> [w170]
            }
            n63 = Number To Decimal String(number=w164, width (-)=3) -> (decimal integer string=w162:string[])
            n64 = case shown="1" w168 {
              tunnel: ["First index (below) pertains to all files " "Indices (below) pertain to each file"] -> w167
              frame 0, Default {
              }
              frame 1 {
              }
            }
            "?" <- w167
            n65 = case shown="True" w161 {
              frame False {
              }
              frame True {
                n66 = property on="mode" class="Bool (strict)"("Val(Sgnl)"=FALSE) -> ()  [unwired: 2 in, 2 out]
              }
            }
            "time interval" <- w166
            "time interval" <- w166
            "time interval" <- w166
          }
          frame #1 {
            n67 = for {
              tunnel: w176 -> [w181]
              tunnel: w175 -> [w180]
              tunnel: w174 -> [w178] mode=indexing
              tunnel: [w179] -> w173 mode=indexing
              n68 = call "tmdsverify.vi"("file path"=w178) -> ("Boolean"=w177:bool)  [unwired: 10 in]
              n69 = stacked-sequence {
                tunnel: w181 -> [w194]
                tunnel: w180 -> [w192]
                tunnel: w178 -> [w185]
                tunnel: [w186] -> w179
                tunnel: w177 -> [w182]
                frame #0 {
                  n70 = Equal?(x=w194, y=1) -> (x = y?=w190:bool)
                  n71 = Equal?(x=w192, y=0) -> (x = y?=w189:bool)
                  n72 = Empty String/Path?(string/path=w185) -> (empty?=w187:bool)
                  n73 = Compound Arithmetic op=AND(w190, w189) -> (w188:bool)
                  n74 = case shown="True" w188 {
                    tunnel: ["" w201] -> w186
                    tunnel: w187 -> [_ w200]
                    tunnel: w185 -> [_ w199]
                    tunnel: "?" -> [_ w198]
                    tunnel: "?" -> [_ w197]
                    tunnel: w182 -> [_ w196]
                    frame False {
                    }
                    frame True {
                      n75 = case shown="False" w200 {
                        tunnel: [w206 ""] -> w201
                        tunnel: w199 -> [w205 _]
                        tunnel: w198 -> [w204 _]
                        tunnel: w197 -> [w203 _]
                        tunnel: w196 -> [w202 _]
                        frame False {
                          n76 = case shown="True" w202 {
                            tunnel: [w210 w220] -> w206
                            tunnel: w205 -> [w209 w221]
                            tunnel: w204 -> [w208 _]
                            tunnel: w203 -> [w207 _]
                            frame False {
                              n77 = case shown="True" w208 {
                                tunnel: [w212 w218] -> w210
                                tunnel: w209 -> [w211 w217]
                                tunnel: w207 -> [_ w215]
                                frame False {
                                n78 = Read from Text File(file (use dialog)=w211) -> (text=w212:string)  [unwired: 2 in, 4 out]
                                }
                                frame True {
                                n79 = Get File Size(file=w217) -> (size (in bytes)=w216:i64)  [unwired: 1 in, 2 out]
                                n80 = In Range and Coerce(upper limit=w216, x=w215, lower limit=0) -> (coerced(x)=w213:u64)  [unwired: 1 out]
                                n81 = Read from Text File(file (use dialog)=w217, count=w213) -> (text=w218:string)  [unwired: 1 in, 4 out]
                                }
                              }
                            }
                            frame True {
                              n82 = call "TDMSchannellist.vi"("file path"=w221) -> ("channel list"=w220:string, "group"=→"Group name":string)  [unwired: 8 in, 1 out]
                            }
                          }
                        }
                        frame True {
                        }
                      }
                    }
                  }
                }
              }
            }
            "file contents" <- w173
          }
          frame #2 {
            n83 = case shown="False" "?" {
              tunnel: "pretrigger time for integration" -> [w254 _]
              tunnel: "pretrigger time for integration" -> [w253 _]
              tunnel: "pretrigger time for integration" -> [_ w255]
              tunnel: [w254 w255] -> w230
              tunnel: [w253 w255] -> w229
              frame False {
              }
              frame True {
              }
            }
            n84 = Bundle("time column selection"="time column selection", "dB/dt column selection"="dB/dt column selection", "B column selection"="B column selection", "data column selection"="data column selection", "data column selection"="data column selection") -> (w244:T13)  [unwired: 1 out]
            n85 = Bundle("pretrigger time for integration"="pretrigger time for integration", "pretrigger time for integration"=w230, "pretrigger time for integration"=w229) -> (w235:T14)  [unwired: 1 out]
            n86 = Bundle("time column rescale"="time column rescale", "dB/dt column rescale"="dB/dt column rescale", "B column rescale"="B column rescale", "data column rescale"="data column rescale", "data column rescale"="data column rescale") -> (w243:T15)  [unwired: 1 out]
            n87 = case shown="False" "?" {
              tunnel: "angle theta (cos theta renorm.)" -> [w249 w252]
              tunnel: [w249 w250] -> w225
              frame False {
              }
              frame True {
                n88 = Multiply(x=w252, y=0) -> (x*y=w250:ext[])
              }
            }
            n89 = Bundle("B column offset"="B column offset", "data column offset"="data column offset", "data column offset"="data column offset") -> (w239:T16)  [unwired: 1 out]
          }
          frame #3 {
            n90 = case shown="True" w257 {
              tunnel: w258 -> [_ w268]
              tunnel: w256 -> [_ w267]
              frame False {
              }
              frame True {
                n91 = for {
                  tunnel: w268 -> [w269] mode=indexing
                  tunnel: [w269] -> _ mode=indexing
                  tunnel: [w271] -> w260 mode=indexing
                  tunnel: [w270] -> w262 mode=indexing
                  n92 = Strip Path(path=w269) -> (stripped path=w270:path, name=w271:string)
                }
                n93 = global write "status.vi" "String"("importing") -> ()
                n94 = Build Path(base path=w267, name or relative path="files") -> (appended path=w264:path)
                n95 = Build Path(base path=w267, name or relative path="paths") -> (appended path=w263:path)
                n96 = Path To String(path=w262) -> (string=w261:string[])
                n97 = call-poly <vilib>:"Write To Spreadsheet File.vi"("1D data"=w260, "file path (dialog if empty)"=w264) -> ()  [unwired: 4 in, 3 out]
                n98 = call-poly <vilib>:"Write To Spreadsheet File.vi"("1D data"=w261, "file path (dialog if empty)"=w263) -> ()  [unwired: 4 in, 3 out]
              }
            }
          }
          frame #4 {
            n99 = Build Array("indx", "time", "bdot", "bcol", "dat1", "dat2") -> (w272:string[])
          }
          frame #5 {
            n100 = Build Path(base path=w279, name or relative path="files") -> (appended path=w284:path)
            n101 = Build Path(base path=w279, name or relative path="paths") -> (appended path=w283:path)
            n102 = call-poly <vilib>:"Read From Spreadsheet File.vi"("file path (dialog if empty)"=w284) -> ("first row"=w282:string[])  [unwired: 3 in, 7 out]
            n103 = call-poly <vilib>:"Read From Spreadsheet File.vi"("file path (dialog if empty)"=w283) -> ("first row"=w281:string[])  [unwired: 3 in, 7 out]
            n104 = String To Path(string=w281) -> (path=w280:path[])
          }
          frame #6 {
            # "create empty binary files"
            n105 = Build Array (concatenate)(w291, "datm") -> (w289:string[])
            n106 = stacked-sequence {
              tunnel: w293 -> [w296 w307]
              tunnel: w292 -> [w295 w305]
              tunnel: w289 -> [w294 w306]
              tunnel: w288 -> [_ w303]
              tunnel: w287 -> [_ w304]
              frame #0 {
                n107 = for {
                  tunnel: w296 -> [_] mode=indexing
                  tunnel: w294 -> [w299]
                  tunnel: w295 -> [w297]
                  i -> [w298]
                  n108 = for {
                    tunnel: w299 -> [w302] mode=indexing
                    tunnel: w298 -> [w301]
                    tunnel: w297 -> [w300]
                    n109 = call "createemptybinary.vi"("base path"=w300, "file index"=w301, "data column"=w302) -> ()  [unwired: 9 out]
                  }
                }
              }
              frame #1 {
                n110 = Equal?(x=w304, y=w303) -> (x = y?=w308:bool)
                n111 = case shown="False" w308 {
                  tunnel: w307 -> [w313 _]
                  tunnel: w306 -> [w312 _]
                  tunnel: w305 -> [w311 _]
                  tunnel: w304 -> [w310 _]
                  tunnel: w303 -> [w309 _]
                  frame False {
                    n112 = for {
                      tunnel: w313 -> [_] mode=indexing
                      tunnel: w312 -> [w318]
                      tunnel: w311 -> [w316]
                      tunnel: w310 -> [w315]
                      tunnel: w309 -> [w314]
                      i -> [w317]
                      n113 = for {
                        tunnel: w318 -> [w321] mode=indexing
                        tunnel: w317 -> [w320]
                        tunnel: w316 -> [w319]
                        tunnel: w315 -> [w324]
                        tunnel: w314 -> [w322]
                        n114 = call "readbinary.vi"(7:w324, "base path"=w319, "file index"=w320, "data column"=w321) -> ("data"=w323:ext[])  [unwired: 7 out]
                        n115 = call "writebinary.vi"(7:w322, "base path"=w319, "file index"=w320, "data column"=w321, "data"=w323) -> ()  [unwired: 7 out]
                      }
                    }
                  }
                  frame True {
                  }
                }
              }
            }
          }
          frame #7 {
            n116 = stacked-sequence {
              tunnel: dbl[] [] ("Array 24") -> [w327 w329 w332 w336 w339]
              frame #0 {
                # "time"
                n117 = case shown="False" "clear arrays" {
                  tunnel: w327 -> [_ w328]
                  frame False {
                  }
                  frame True {
                    n118 = property on="time column selection" class="Arr (strict)"("Val(Sgnl)"=w328) -> ()  [unwired: 2 in, 2 out]
                    n119 = property on="time column rescale" class="Arr (strict)"("Val(Sgnl)"=w328) -> ()  [unwired: 2 in, 2 out]
                  }
                }
              }
              frame #1 {
                # "dB/dt"
                n120 = case shown="True" "clear arrays" {
                  tunnel: w329 -> [_ w331]
                  frame False {
                  }
                  frame True {
                    n121 = property on="dB/dt column rescale" class="Arr (strict)"("Val(Sgnl)"=w331) -> ()  [unwired: 2 in, 2 out]
                    n122 = property on="dB/dt column selection" class="Arr (strict)"("Val(Sgnl)"=w331) -> ()  [unwired: 2 in, 2 out]
                  }
                }
              }
              frame #2 {
                # "field"
                n123 = case shown="True" "clear arrays" {
                  tunnel: w332 -> [_ w334]
                  frame False {
                  }
                  frame True {
                    n124 = local write "B column selection"(w334) -> ()
                    n125 = property on="B column rescale" class="Arr (strict)"("Val(Sgnl)"=w334) -> ()  [unwired: 2 in, 2 out]
                    n126 = property on="angle theta (cos theta renorm.)" class="Arr (strict)"("Val(Sgnl)"=w334) -> ()  [unwired: 2 in, 2 out]
                    n127 = property on="B column offset" class="Arr (strict)"("Val(Sgnl)"=w334) -> ()  [unwired: 2 in, 2 out]
                  }
                }
              }
              frame #3 {
                # "data1"
                n128 = case shown="False" "clear arrays" {
                  tunnel: w336 -> [_ w337]
                  frame False {
                  }
                  frame True {
                    n129 = property on="data column rescale" class="Arr (strict)"("Val(Sgnl)"=w337) -> ()  [unwired: 2 in, 2 out]
                    n130 = property on="data column offset" class="Arr (strict)"("Val(Sgnl)"=w337) -> ()  [unwired: 2 in, 2 out]
